vi "Find Compatible AVI Files.vi"(3 "Video Path":path) -> (0 "RGB Path":path, 1 "Depth Path":path)   [LabVIEW 2018]
uses:
  <vilib>/regexp/Match Regular Expression.xnode
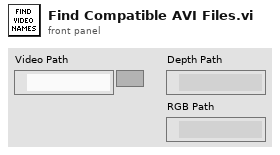
[diagram p1: front panel]
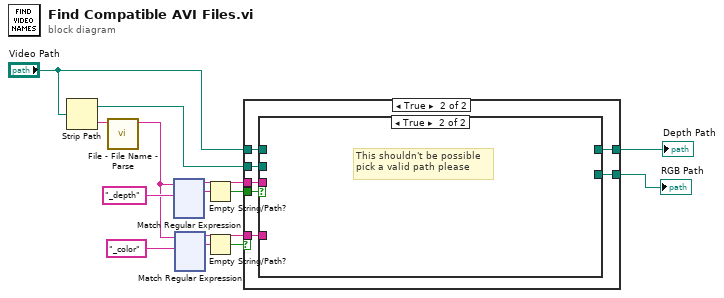
[diagram p0: block diagram]
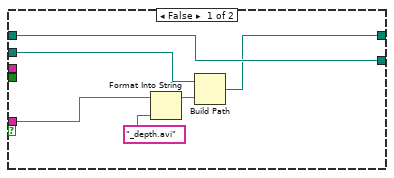
[diagram p2: hidden frame]
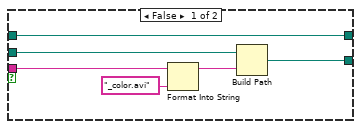
[diagram p3: hidden frame]
diagram:
  n1 = Strip Path(path="Video Path") -> (stripped path=w6:path, name=w14:string)
  n2 = call <userlib>:"File - File Name - Parse.vi"("File Name"=w14) -> ("Base Name"=w12:string)  [unwired: 8 in, 2 out]
  n3 = xnode "Match Regular Expression"("input string"=w12, "regular expression"="_depth") -> ("before match"=w3:string, "whole match"=w10:string)  [unwired: 4 in, 3 out]
  n4 = xnode "Match Regular Expression"("input string"=w12, "regular expression"="_color") -> ("before match"=w2:string, "whole match"=w8:string)  [unwired: 4 in, 3 out]
  n5 = Empty String/Path?(string/path=w10) -> (empty?=w7:bool)
  n6 = Empty String/Path?(string/path=w8) -> (empty?=w9:bool)
  n7 = case shown="True" w9 {
    tunnel: w7 -> [_ w27]
    tunnel: w6 -> [w19 w26]
    tunnel: "Video Path" -> [w20 w25]
    tunnel: [w15 w24] -> w4
    tunnel: w3 -> [_ w23]
    tunnel: w2 -> [w17 w22]
    tunnel: [w20 w21] -> w1
    frame False {
      n8 = Format Into String(initial string=w17, "_depth.avi") -> (resulting string=w18:string)  [unwired: 2 in, 1 out]
      n9 = Build Path(base path=w19, name or relative path=w18) -> (appended path=w15:path)
    }
    frame True {
      n10 = case shown="True" w27 {
        tunnel: w26 -> [w32 _]
        tunnel: w25 -> [w33 _]
        tunnel: [w33 _] -> w24
        tunnel: w23 -> [w31 _]
        tunnel: w22 -> [_ _]
        tunnel: [w28 _] -> w21
        frame False {
          n11 = Format Into String(initial string=w31, "_color.avi") -> (resulting string=w30:string)  [unwired: 2 in, 1 out]
          n12 = Build Path(base path=w32, name or relative path=w30) -> (appended path=w28:path)
        }
        frame True {
          # "This shouldn't be possible\npick a valid path please"
        }
      }
    }
  }
  "Depth Path" <- w4
  "RGB Path" <- w1
